vi "2 station_keeping_points.vi"(9 "Which Point?":i32, 10 "Midpoint":T1 {"North" format="%#_10f"; "East" format="%#_8f"}) -> (2 "Waypoint":T1 {"North" format="%#_10f"; "East" format="%#_8f"})   [LabVIEW 2011]
uses:
  2 Typedefs/UTM Location.ctl
  2 Typedefs/absolute wind direction.ctl
  2 Globals/2 Global.vi
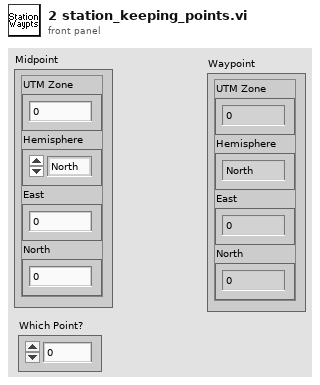
[diagram p1: front panel]
types:
  T1 = typedef "UTM Location.ctl" = cluster{"UTM Zone":dbl, "Hemisphere":enum16{"North", "South"}, "East":dbl, "North":dbl}
  T2 = typedef "absolute wind direction.ctl" = dbl
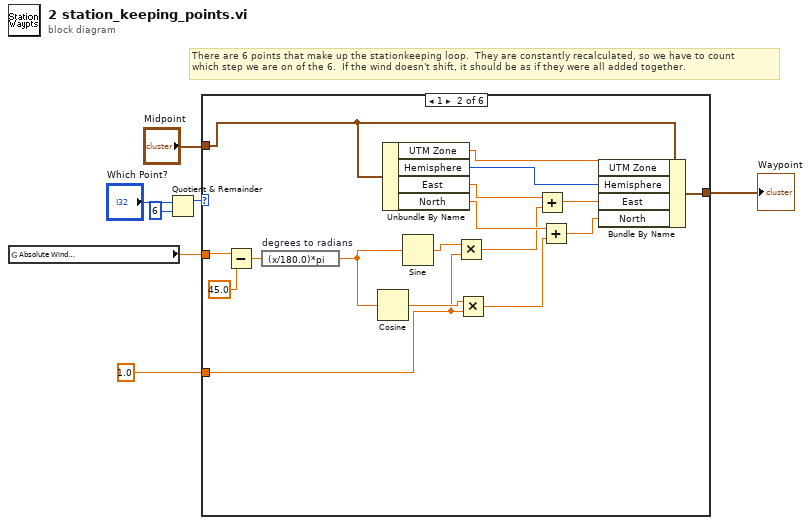
[diagram p0: block diagram]
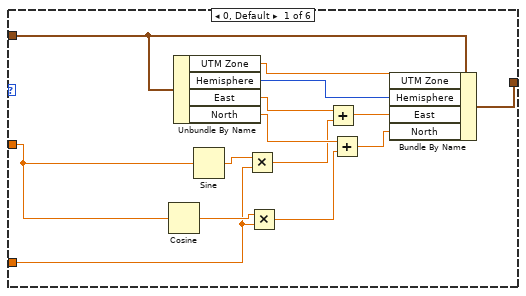
[diagram p2: hidden frame]
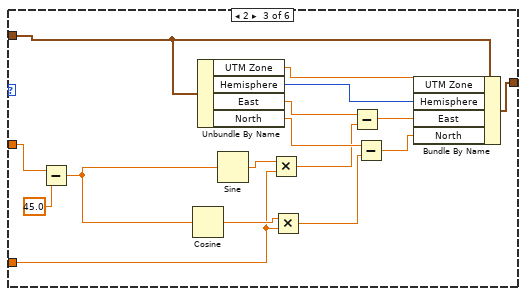
[diagram p3: hidden frame]
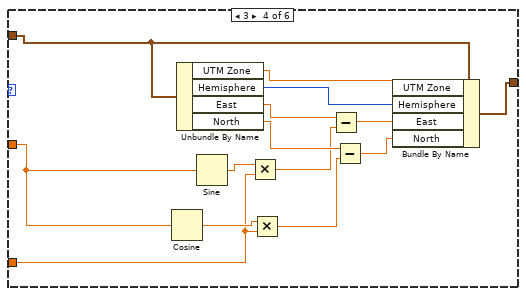
[diagram p4: hidden frame]
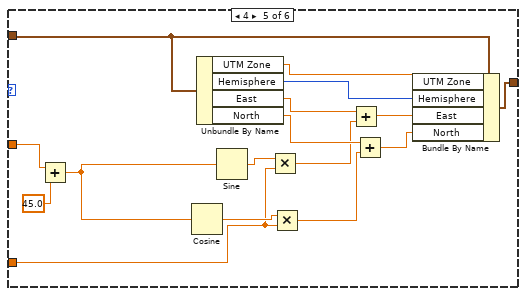
[diagram p5: hidden frame]
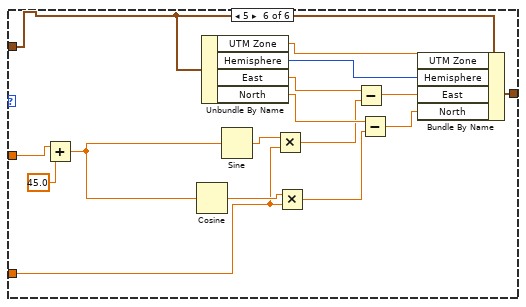
[diagram p6: hidden frame]
diagram:
  # "There are 6 points that make up the stationkeeping loop.  They are constantly recalculated, so we have to count\nwhich step we are on of the 6.  If the wind doesn't shift, it should be as if they were all added together."
  n1 = global read "2 Global.vi" "Absolute Wind\nDirection (º)"() -> (w3:T2)
  n2 = Quotient & Remainder(x="Which Point?", y=6) -> (x-y*floor(x/y)=w5:i32)  [unwired: 1 out]
  n3 = case shown="1" w5 {
    tunnel: "Midpoint" -> [w20 w27 w41 w57 w71 w87]
    tunnel: w3 -> [w9 w26 w40 w56 w70 w86]
    tunnel: [w21 w28 w42 w58 w72 w88] -> w2
    tunnel: T2 1.0 ("y") -> [w8 w24 w39 w55 w69 w85]
    frame 0, Default {
      n4 = Cosine(x=w9) -> (cos(x)=w16:T2)
      n5 = Unbundle By Name(w20) -> ("UTM Zone"=w19:dbl, "Hemisphere"=w18:enum16{"North", "South"}, "East"=w14:dbl, "North"=w12:dbl)
      n6 = Sine(x=w9) -> (sin(x)=w17:T2)
      n7 = Multiply(x=w17, y=w8) -> (x*y=w11:T2)
      n8 = Multiply(x=w16, y=w8) -> (x*y=w10:T2)
      n9 = Add(x=w14, y=w11) -> (x+y=w15:T2)
      n10 = Add(x=w12, y=w10) -> (x+y=w13:T2)
      n11 = Bundle By Name(cluster=w20, "UTM Zone"=w19, "Hemisphere"=w18, "East"=w15, "North"=w13) -> (w21:T1)
    }
    frame 1 {
      n12 = Subtract(x=w26, y=T2 45.0) -> (x-y=w23:T2)
      n13 = expression code="(x/180.0)*pi" "degrees to radians"(w23) -> (w22:T2)
      n14 = Cosine(x=w22) -> (cos(x)=w35:T2)
      n15 = Unbundle By Name(w27) -> ("UTM Zone"=w38:dbl, "Hemisphere"=w37:enum16{"North", "South"}, "East"=w33:dbl, "North"=w31:dbl)
      n16 = Sine(x=w22) -> (sin(x)=w36:T2)
      n17 = Multiply(x=w36, y=w24) -> (x*y=w30:T2)
      n18 = Multiply(x=w35, y=w24) -> (x*y=w29:T2)
      n19 = Add(x=w33, y=w30) -> (x+y=w34:T2)
      n20 = Add(x=w31, y=w29) -> (x+y=w32:T2)
      n21 = Bundle By Name(cluster=w27, "UTM Zone"=w38, "Hemisphere"=w37, "East"=w34, "North"=w32) -> (w28:T1)
    }
    frame 2 {
      n22 = Subtract(x=w40, y=T2 45.0) -> (x-y=w44:T2)
      n23 = Cosine(x=w44) -> (cos(x)=w51:T2)
      n24 = Unbundle By Name(w41) -> ("UTM Zone"=w54:dbl, "Hemisphere"=w53:enum16{"North", "South"}, "East"=w49:dbl, "North"=w47:dbl)
      n25 = Sine(x=w44) -> (sin(x)=w52:T2)
      n26 = Multiply(x=w52, y=w39) -> (x*y=w46:T2)
      n27 = Multiply(x=w51, y=w39) -> (x*y=w45:T2)
      n28 = Subtract(x=w49, y=w46) -> (x-y=w50:T2)
      n29 = Subtract(x=w47, y=w45) -> (x-y=w48:T2)
      n30 = Bundle By Name(cluster=w41, "UTM Zone"=w54, "Hemisphere"=w53, "East"=w50, "North"=w48) -> (w42:T1)
    }
    frame 3 {
      n31 = Cosine(x=w56) -> (cos(x)=w65:T2)
      n32 = Unbundle By Name(w57) -> ("UTM Zone"=w68:dbl, "Hemisphere"=w67:enum16{"North", "South"}, "East"=w63:dbl, "North"=w61:dbl)
      n33 = Sine(x=w56) -> (sin(x)=w66:T2)
      n34 = Multiply(x=w66, y=w55) -> (x*y=w60:T2)
      n35 = Multiply(x=w65, y=w55) -> (x*y=w59:T2)
      n36 = Subtract(x=w63, y=w60) -> (x-y=w64:T2)
      n37 = Subtract(x=w61, y=w59) -> (x-y=w62:T2)
      n38 = Bundle By Name(cluster=w57, "UTM Zone"=w68, "Hemisphere"=w67, "East"=w64, "North"=w62) -> (w58:T1)
    }
    frame 4 {
      n39 = Add(x=w70, y=T2 45.0) -> (x+y=w74:T2)
      n40 = Cosine(x=w74) -> (cos(x)=w81:T2)
      n41 = Unbundle By Name(w71) -> ("UTM Zone"=w84:dbl, "Hemisphere"=w83:enum16{"North", "South"}, "East"=w79:dbl, "North"=w77:dbl)
      n42 = Sine(x=w74) -> (sin(x)=w82:T2)
      n43 = Multiply(x=w82, y=w69) -> (x*y=w76:T2)
      n44 = Multiply(x=w81, y=w69) -> (x*y=w75:T2)
      n45 = Add(x=w79, y=w76) -> (x+y=w80:T2)
      n46 = Add(x=w77, y=w75) -> (x+y=w78:T2)
      n47 = Bundle By Name(cluster=w71, "UTM Zone"=w84, "Hemisphere"=w83, "East"=w80, "North"=w78) -> (w72:T1)
    }
    frame 5 {
      n48 = Add(x=w86, y=T2 45.0) -> (x+y=w90:T2)
      n49 = Cosine(x=w90) -> (cos(x)=w97:T2)
      n50 = Unbundle By Name(w87) -> ("UTM Zone"=w100:dbl, "Hemisphere"=w99:enum16{"North", "South"}, "East"=w95:dbl, "North"=w93:dbl)
      n51 = Sine(x=w90) -> (sin(x)=w98:T2)
      n52 = Multiply(x=w98, y=w85) -> (x*y=w92:T2)
      n53 = Multiply(x=w97, y=w85) -> (x*y=w91:T2)
      n54 = Subtract(x=w95, y=w92) -> (x-y=w96:T2)
      n55 = Subtract(x=w93, y=w91) -> (x-y=w94:T2)
      n56 = Bundle By Name(cluster=w87, "UTM Zone"=w100, "Hemisphere"=w99, "East"=w96, "North"=w94) -> (w88:T1)
    }
  }
  "Waypoint" <- w2
